vi "isComplete.vi"(8 "error in (no error)":errorcluster, 11 "Mission in":refnum<class "Idle.lvclass">) -> (0 "error out":errorcluster, 2 "Mission Complete?":bool, 3 "Mission out":refnum<class "Idle.lvclass">)   [LabVIEW 2011, in "Idle.lvclass"]
doc: "Determine whether or not a mission is complete.\n\nIn this case, it is complete when a mission is added to the queue. When it completes, it deletes the waypoint it added on start.\n\nNote: This is a dynamic dispatch method of GenericMission. The correct method will be called based on the run-time class of this object, a child class of GenericMission.\n\nAuthor: Jared Kirschner"
uses:
  Idle.lvclass
  MissionQueue/MissionQueue.lvclass
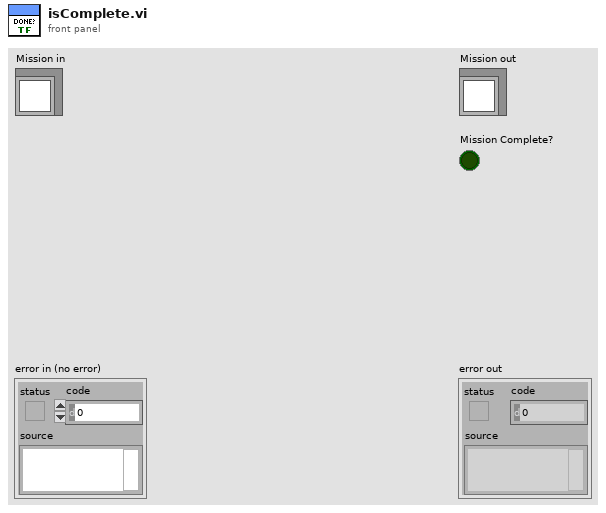
[diagram p1: front panel]
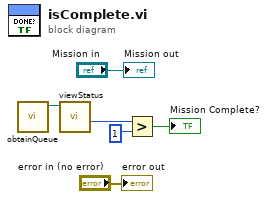
[diagram p0: block diagram]
diagram:
  n1 = call "obtainQueue.vi"() -> ("MissionQueue.lvclass"=w5:refnum<class "MissionQueue.lvclass">)  [unwired: 10 in, 1 out]
  n2 = call "viewStatus.vi"("MissionQueue in"=w5) -> ("Queue length"=w4:i32)  [unwired: 6 in, 4 out]
  n3 = Greater?(x=w4, y=1) -> (0:→"Mission Complete?":bool)
  "error out" <- "error in (no error)"
  "Mission out" <- "Mission in"
